vi "Draw_rectangle_oval.vi"() -> ()   [LabVIEW 2023]
panel:
  out "Canvas":picture
  in  "stop":bool
  in  "Datos Rectangulo":T1
  in  "Datos Ovalo":T1
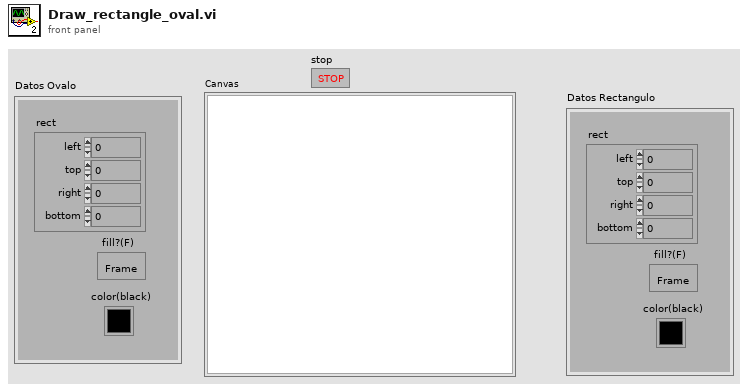
[diagram p1: front panel]
types:
  T1 = cluster{"rect":cluster{"left":i16, "top":i16, "right":i16, "bottom":i16}, "fill?(F)":bool, "color(black)":u32}
  T2 = cluster{"left":i16, "top":i16, "right":i16, "bottom":i16}
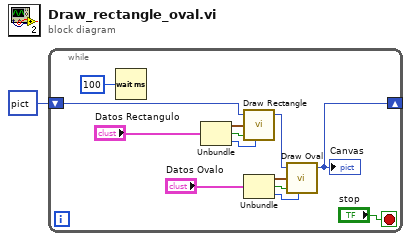
[diagram p0: block diagram]
diagram:
  n1 = while {
    shift-right: [w2] -> _
    shift-left: picture data[5B] ("picture") -> [w3]
    stop <- "stop" stop-if-true
    n2 = Wait (ms)(milliseconds to wait=u32 100 ("millisecond timer value")) -> ()  [unwired: 1 out]
    n3 = Unbundle("Datos Rectangulo") -> ("rect"=w11:T2, "fill?(F)"=w10:bool, "color(black)"=w9:u32)
    n4 = call <vilib>:"Draw Rectangle.vi"("picture"=w3, "rect"=w11, "fill?(F)"=w10, "color(black)"=w9) -> ("new picture"=w8:picture)  [unwired: 5 in]
    n5 = Unbundle("Datos Ovalo") -> ("rect"=w6:T2, "fill?(F)"=w5:bool, "color(black)"=w4:u32)
    n6 = call <vilib>:"Draw Oval.vi"("picture"=w8, "rect"=w6, "fill?(F)"=w5, "color(black)"=w4) -> ("new picture"=w2:picture)  [unwired: 5 in]
    "Canvas" <- w2
  }
